vi "SetIOPinDly.vi"(8 "错误输入（无错误）":errorcluster, 10 "闸门跟踪属性":u16) -> (0 "错误输出":errorcluster)   [LabVIEW 2014]
uses:
  X86Dll/ZXUTConfigMgr.dll
panel:
  in  "SelPinType":i32
  in  "SelPinNum":i32
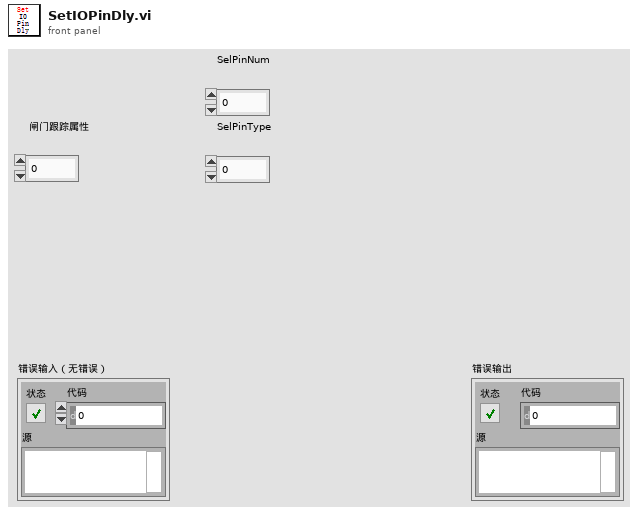
[diagram p1: front panel]
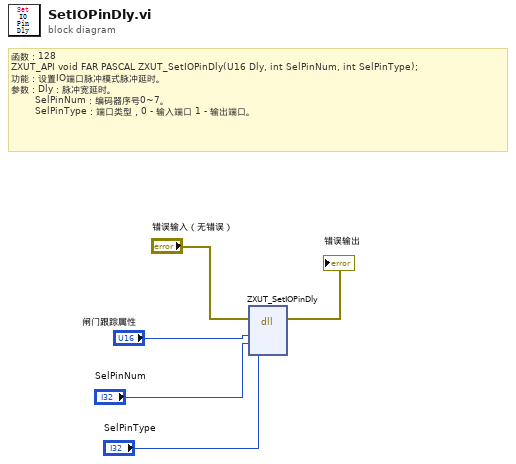
[diagram p0: block diagram]
diagram:
  # "函数：128\nZXUT_API void\tFAR PASCAL ZXUT_SetIOPinDly(U16 Dly, int SelPinNum, int SelPinType);\n功能：设置IO端口脉冲模式脉冲延时。\n参数：Dly：脉冲宽延时。\n        SelPinNum：编码器序号0~7。\n        SelPinType：端口类型，0 - 输入端口 1 - 输出端口。"
  n1 = dll-call lib="D:/Software/Utrasonic on-line monitoring/X86Dll/ZXUTConfigMgr.dll" fn="ZXUT_SetIOPinDly"(error in="错误输入（无错误）", "Dly"="闸门跟踪属性", "SelPinNum"="SelPinNum", "SelPinType"="SelPinType") -> (error out=→"错误输出":errorcluster)  [unwired: 6 in, 1 out]
